vi "Create All Message Queues Camera.vi"(8 "error in (no error)":cluster{"状态":bool, "代码":i32, "源":string} caption="错误输入（无错误）") -> (0 "error out":cluster{"状态":bool, "代码":i32, "源":string} caption="错误输出", 3 "消息队列":T1)   [LabVIEW 2015, in "Message Queue.lvlib"]
doc: "本VI用于创建应用程序所需的所有消息队列。如应用程序需要两个以上消息队列，可右键单击上面的“消息队列”常量并选择打开自定义类型，将新的消息队列添加至该自定义类型，然后通过本VI进行初始化。"
uses:
  Message Queue.lvlib
  All Message Queues Camera.ctl
  Message Cluster.ctl
  Enqueue Message (Single).vi
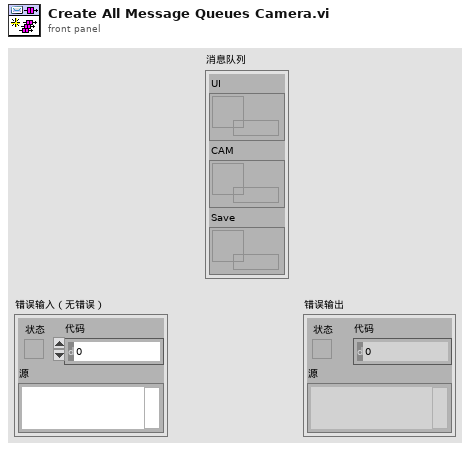
[diagram p1: front panel]
types:
  T1 = typedef "Message Queue.lvlib/All Message Queues Camera.ctl" = cluster{"UI":refnum<queue>, "CAM":refnum<queue>, "Save":refnum<queue>}
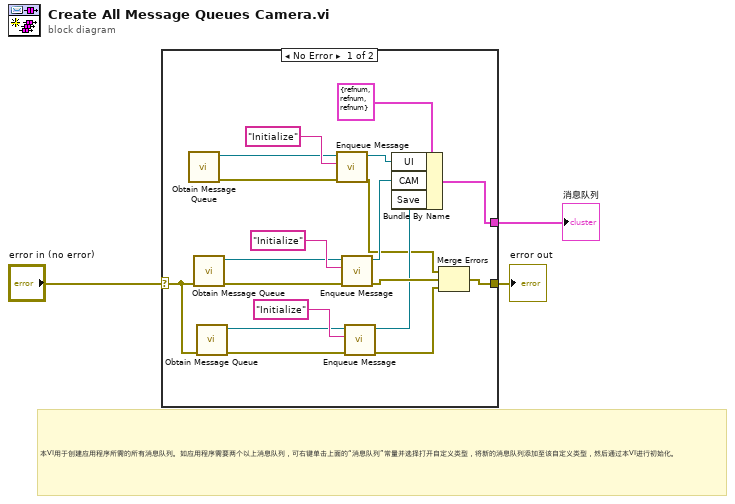
[diagram p0: block diagram]
diagram:
  # "本VI用于创建应用程序所需的所有消息队列。如应用程序需要两个以上消息队列，可右键单击上面的“消息队列”常量并选择打开自定义类型，将新的消息队列添加至该自定义类型，然后通过本VI进行初始化。"
  n1 = case shown="No Error" "error in (no error)" {
    selector: "error in (no error)" -> [w15 w23]
    tunnel: [w14 w23] -> w3
    tunnel: [w22 _] -> w1
    frame No Error {
      n2 = call "Obtain Message Queue.vi"() -> ("error out"=w8:cluster{"状态":bool, "代码":i32, "源":string}, "消息队列"=w6:refnum<queue>)  [unwired: 10 in]
      n3 = call "Obtain Message Queue.vi"("error in (no error)"=w15) -> ("error out"=w21:cluster{"状态":bool, "代码":i32, "源":string}, "消息队列"=w19:refnum<queue>)  [unwired: 9 in]
      n4 = call "Obtain Message Queue.vi"("error in (no error)"=w15) -> ("error out"=w18:cluster{"状态":bool, "代码":i32, "源":string}, "消息队列"=w16:refnum<queue>)  [unwired: 9 in]
      n5 = call-poly "Enqueue Message.vi"("error in (no error)"=w8, "消息"="Initialize" ("Message"), "消息队列"=w6) -> ("error out"=w4:cluster{"状态":bool, "代码":i32, "源":string}, "消息队列副本"=w5:refnum<queue>)  [unwired: 7 in]
      n6 = call-poly "Enqueue Message.vi"("error in (no error)"=w21, "消息"="Initialize" ("Message"), "消息队列"=w19) -> ("error out"=w13:cluster{"状态":bool, "代码":i32, "源":string}, "消息队列副本"=w10:refnum<queue>)  [unwired: 7 in]
      n7 = call-poly "Enqueue Message.vi"("error in (no error)"=w18, "消息"="Initialize" ("Message"), "消息队列"=w16) -> ("error out"=w12:cluster{"状态":bool, "代码":i32, "源":string}, "消息队列副本"=w11:refnum<queue>)  [unwired: 7 in]
      n8 = Bundle By Name(cluster=T1 {"UI"=refnum, "CAM"=refnum, "Save"=refnum} ("消息队列"), "UI"=w5, "CAM"=w10, "Save"=w11) -> (w22:T1)
      n9 = Merge Errors(w4, w13, w12) -> (w14:errorcluster)
    }
    frame Error {
    }
  }
  "error out" <- w3
  "消息队列" <- w1
